vi "ModbusWithThread.vi"() -> ()   [LabVIEW 2014]
uses:
  <vilib>/Platform/TimedLoop/XDataNode/timing_clust.ctl
  <vilib>/Platform/TimedLoop/XDataNode/nitl_modes.ctl
  <vilib>/Platform/TimedLoop/XDataNode/wakeup.ctl
  globalTestRasp.vi
  ModbusLibHMI/compareArrayDataCoil.vi
  ModbusLibHMI/compareArrayDataHold.vi
  <vilib>/platform/TimedLoop/XDataNode/XDataNode.xnode
  <vilib>/Platform/TimedLoop/XDataNode/XDNodeRunTimeDep.lvlib
panel:
  out "Value":u16
  in  "error in (no error)":errorcluster
  out "CoilChange":bool[](array[boolean])
  out "HoldingChange":u16[](array[numeric])
  in  "stop":bool
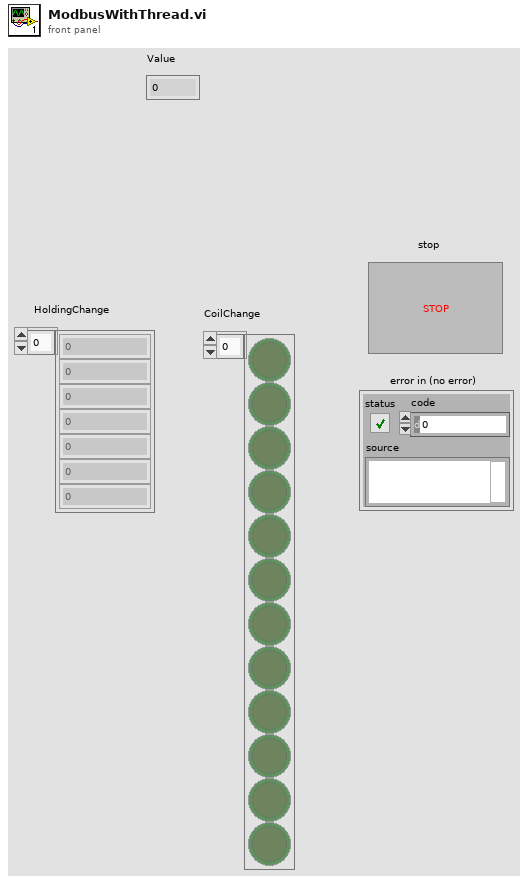
[diagram p1: front panel]
types:
  T1 = cluster{"eventCoil":refnum<user-event>, "eventHold":refnum<user-event>}
  T2 = typedef "XDNodeRunTimeDep.lvlib/timing_clust.ctl" = cluster{"Expected End [f-1]":u64, "Actual End [f-1]":u64, "Finished Late? [f-1]":bool, "Expected End [i-1]":u64, "Actual End [i-1]":u64, "Finished Late? [i-1]":bool, "Expected Start [i]":u64, "Actual Start [i]":u64, "Expected Start [f]":u64, "Actual Start [f]":u64, "Source Name":string, "Structure Name":string, "Period":i64, "Deadline":i64, "Offset":i64, "Start":i64, "Priority":i32, "Timeout":i32, "Mode":T3, "Wakeup Reason":T4, "Error":errorcluster, "Source Type":string, "Secondary Source Type":string, "Global End Time":u64, "Global Start Time":u64, "Frame Duration":u64, "Iteration Duration":u64, "Assigned CPU":i32, "I/O Scan Engine Mode":u32}
  T3 = typedef "XDNodeRunTimeDep.lvlib/nitl_modes.ctl" = enum32{"No Change", "Process missed periods, maintain original phase", "Discard missed periods, maintain original phase", "Process missed periods, ignore original phase", "Discard missed periods, ignore original phase"}
  T4 = typedef "XDNodeRunTimeDep.lvlib/wakeup.ctl" = enum32{"Normal", "Aborted", "Asynchronous wakeup", "Timing source error", "Timed loop error", "Timeout"}
  T5 = enum16{"WriteCoil", "WriteHold", "ChangeID", "Stop"}
  T6 = cluster{"StartAddress":u16, "DataHold":u16[], "datacoil":bool, "AddressModbus":u16, "stateCMD":enum16{"WriteCoil", "WriteHold", "ChangeID", "Stop"}}
  T7 = enum16{"NonEvent", "EMG", "X+", "X-", "Y+", "Y-", "Z+", "Z-", "Mode", "GoHome", "StartAuto", "SaveEprom", "SetAccel", "SetFeedRate", "SetStepSize", "SetStartAccel", "ResetError", "AddG0", "AddG1", "AddSoleNoid", "AddPWM", "AddFan", "WaitInput", "AddSpin", "ControlSpin"}
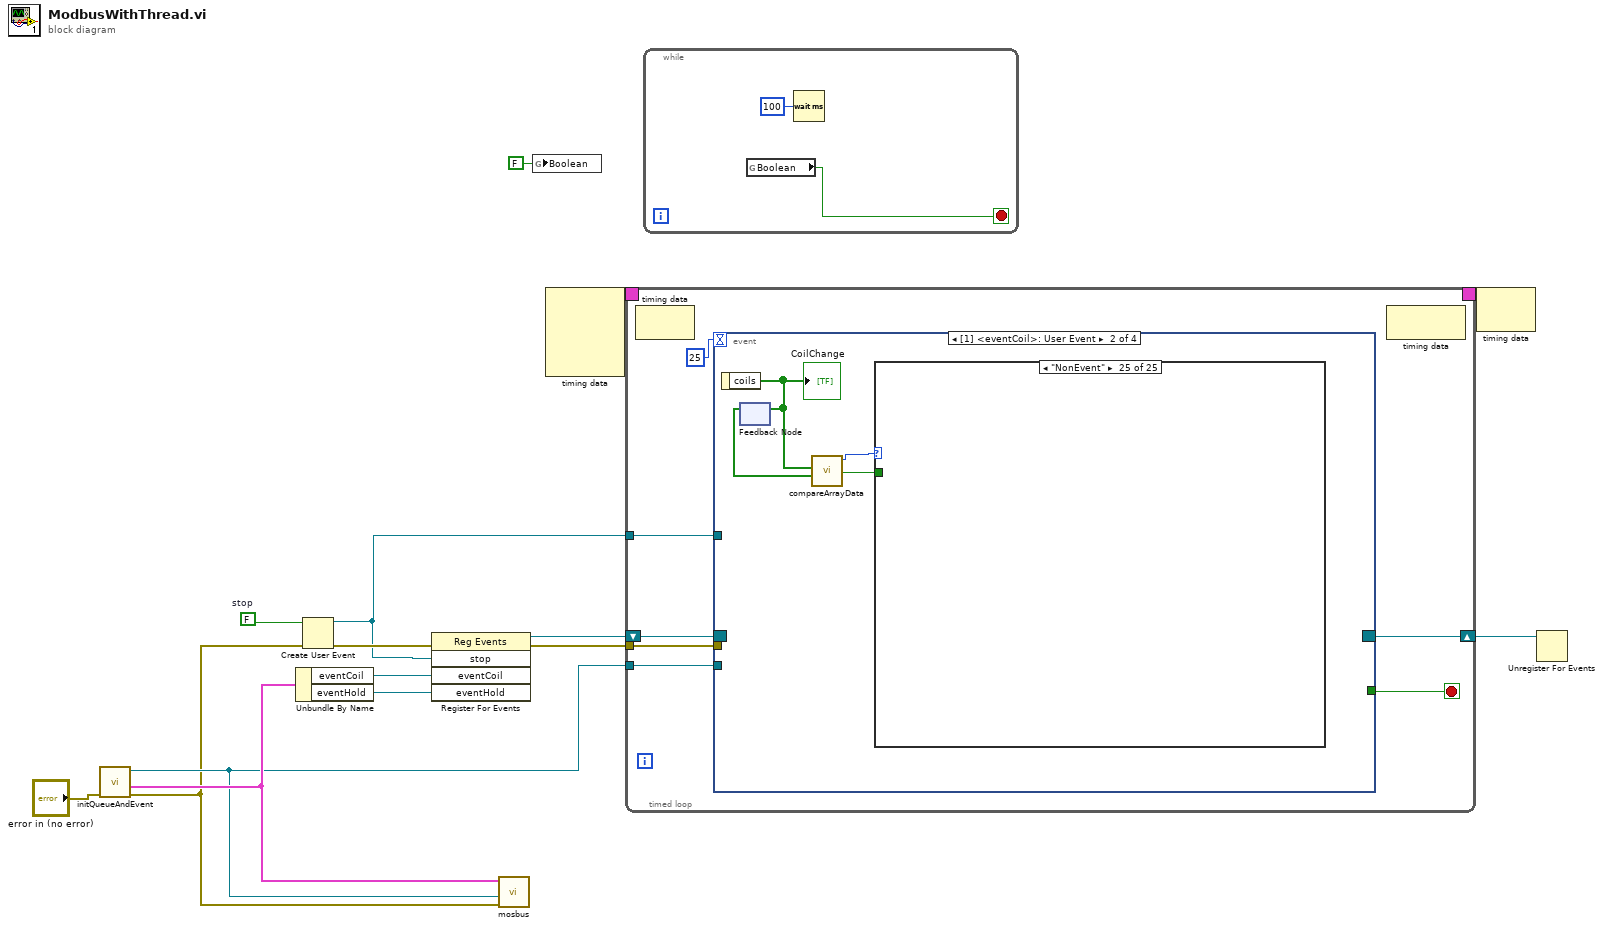
[diagram p0: block diagram]
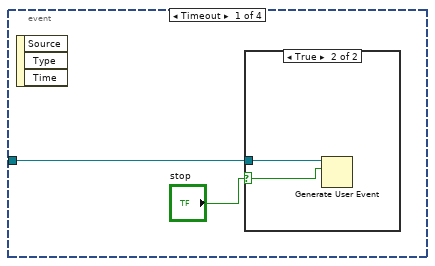
[diagram p2: hidden frame]
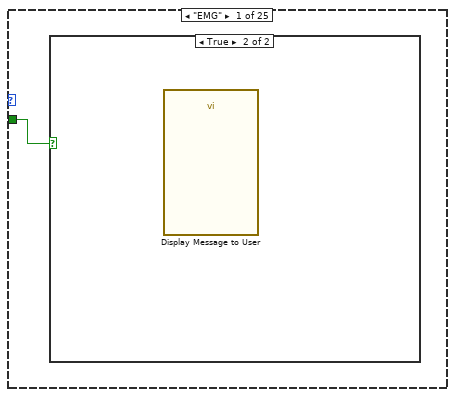
[diagram p4: hidden frame]
diagram:
  w13 = FALSE  # stop
  n1 = call "initQueueAndEvent.vi"("error in (no error)"="error in (no error)") -> ("error out"=w3:errorcluster, "EventOut"=w6:T1, "QueueOut"=w5:refnum<queue>)  [unwired: 8 in]
  n2 = Unbundle By Name(w6) -> ("eventCoil"=w8:refnum<user-event>, "eventHold"=w7:refnum<user-event>)
  n3 = Create User Event(user event datatype=w13, error in=w3) -> (user event=w1:refnum<user-event>, error out=w11:errorcluster)
  n4 = register-events(error in=w11, w1, w8, w7) -> (reference out=w9:refnum<event-registration>, error out=w10:errorcluster)  [unwired: 1 in]
  n5 = call "mosbus.vi"("error in (no error)"=w3, "Queue"=w5, "Event"=w6) -> ()  [unwired: 5 in]
  n6 = global write "globalTestRasp.vi" "Boolean"(FALSE ("Boolean")) -> ()
  n7 = node-c288() -> (w15:T2)  [unwired: 4 in]
  n8 = timed-loop {
    timing: w15 -> [_]
    timing-out: [_] -> w14
    tunnel: w5 -> [w21]
    tunnel: w1 -> [w19]
    shift-right: [w17] -> w12
    shift-left: w9 -> [w22]
    tunnel: w10 -> [w16]
    stop <- w20 stop-if-true
    n9 = node-c288() -> ()  [unwired: 1 in, 1 out]
    n10 = event shown="[1] <eventCoil>: User Event" {
      selector: w22 -> [_ _ _ _]
      dyn-events: [_ _ _ _] -> w17
      timeout: 25 -> [_ _ _ _]
      tunnel: w21 -> [_ _ _ w41]
      tunnel: [_ _ _ TRUE] -> w20
      tunnel: w19 -> [w23 _ _ _]
      tunnel: w16 -> [_ _ _ _]
      event Timeout {
        n11 = event-data() -> ()  [unwired: 1 in, 3 out]
        n12 = case shown="True" "stop" {
          selector: "stop" -> [_ w25]
          tunnel: w23 -> [_ w26]
          frame False {
          }
          frame True {
            n13 = Generate User Event(user event=w26, event data cluster=w25) -> ()  [unwired: 2 in, 2 out]
          }
        }
      }
      event User Event {
        n14 = event-data() -> ("coils"=w29:bool[])  [unwired: 1 in]
        "CoilChange" <- w29
        n15 = feedback-in #1(w29) -> ()
        n16 = feedback #1() -> (w30:bool[])  [unwired: 1 in]
        n17 = call-poly "compareArrayData.vi"("B"=w30, "A"=w29) -> ("Value"=w28:bool, "Enum"=w27:T7)  [unwired: 7 in, 1 out]
        n18 = case shown="\"NonEvent\"" w27 {
          tunnel: w28 -> [w31 _ _ _ _ _ _ _ _ _ _ _ _ _ _ _ _ _ _ _ _ _ _ _ _]
          frame "EMG" {
            n19 = case shown="True" w31 {
              frame False {
              }
              frame True {
                n20 = call "Display Message to User"() -> ()  [unwired: 10 in, 2 out]
              }
            }
          }
          frame "X+" {
          }
          frame "X-" {
          }
          frame "Y+" {
          }
          frame "Y-" {
          }
          frame "Z+" {
          }
          frame "Z-" {
          }
          frame "Mode" {
          }
          frame "GoHome" {
          }
          frame "StartAuto" {
          }
          frame "SaveEprom" {
          }
          frame "SetAccel" {
          }
          frame "SetFeedRate" {
          }
          frame "SetStepSize" {
          }
          frame "SetStartAccel" {
          }
          frame "ResetError" {
          }
          frame "AddG0" {
          }
          frame "AddG1" {
          }
          frame "AddSoleNoid" {
          }
          frame "AddPWM" {
          }
          frame "AddFan" {
          }
          frame "WaitInput" {
          }
          frame "AddSpin" {
          }
          frame "ControlSpin" {
          }
          frame "NonEvent" {
          }
        }
      }
      event User Event {
        n21 = event-data() -> ("register values 3"=w32:u16[])  [unwired: 1 in]
        "HoldingChange" <- w32
        n22 = feedback #2() -> (w33:u16[])  [unwired: 1 in]
        n23 = feedback-in #2(w32) -> ()
        n24 = call-poly "compareArrayData.vi"("B"=w33, "A"=w32) -> ("Value"=w34:u16, "BitChange"=w35:i32)  [unwired: 8 in]
        n25 = case shown="2" w35 {
          tunnel: w34 -> [_ _ w36 _ _]
          frame 0, Default {
          }
          frame 1 {
          }
          frame 2 {
            "Value" <- w36
          }
          frame 3 {
          }
          frame 4 {
          }
        }
      }
      event User Event {
        n26 = event-data() -> ()  [unwired: 1 in, 5 out]
        n27 = Bundle By Name(cluster=T6 {"StartAddress"=0, "DataHold"=[], "datacoil"=FALSE, "AddressModbus"=0, "stateCMD"=enum."Stop"} ("element"), "stateCMD"=T5."Stop") -> (w39:T6)
        n28 = global write "globalTestRasp.vi" "Boolean"(TRUE ("Boolean")) -> ()
        n29 = Enqueue Element(queue=w41, element=w39) -> ()  [unwired: 2 in, 3 out]
      }
    }
    n30 = node-c288() -> ()  [unwired: 1 in, 1 out]
  }
  n31 = while {
    stop <- w46 stop-if-true
    n32 = global read "globalTestRasp.vi" "Boolean"() -> (w46:bool)
    n33 = Wait (ms)(milliseconds to wait=u32 100) -> ()  [unwired: 1 out]
  }
  n34 = node-c288(w14) -> ()  [unwired: 1 out]
  n35 = Unregister For Events(event registration refnum=w12) -> ()  [unwired: 1 in, 1 out]
